vi "Previous Element Sum.vi"() -> ()   [LabVIEW 2019]
panel:
  out "Output Array":dbl[](array[numeric])
  in  "Input Array":dbl[](array[numeric])
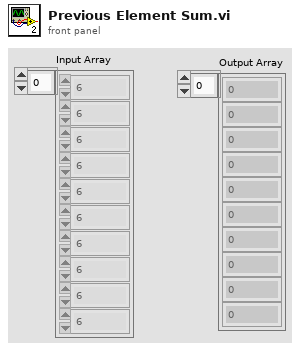
[diagram p1: front panel]
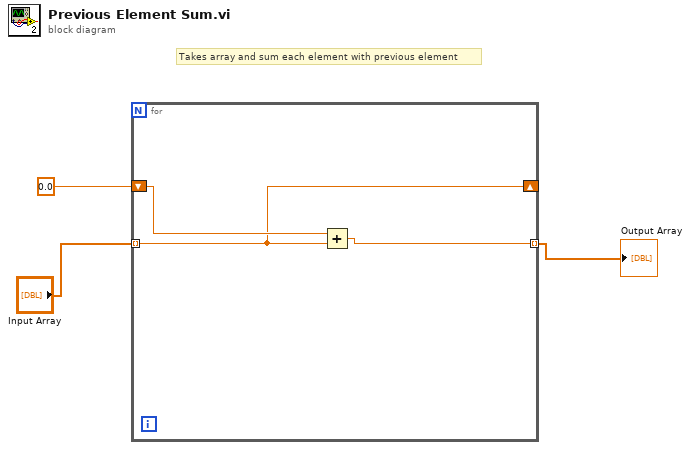
[diagram p0: block diagram]
diagram:
  # "Takes array and sum each element with previous element"
  n1 = for {
    shift-right: [w4] -> _
    shift-left: 0.0 -> [w6]
    tunnel: [w5] -> w1 mode=indexing
    tunnel: "Input Array" -> [w4] mode=indexing
    n2 = Add(x=w6, y=w4) -> (x+y=w5:dbl)
  }
  "Output Array" <- w1
